vi "Run Test (ProjectRefnum).vi"(5 "Test Report":refnum<class "Test Report.lvclass">, 6 "Verbose":bool, 7 "Report Path":path, 8 "error in":errorcluster, 9 "Virtual Folder (My Computer)":string, 10 "Project Refnum":refnum<vi>, 11 "Interactive (T)":bool=TRUE) -> (0 "error out":errorcluster)   [LabVIEW 2013, in "Caraya.lvlib"]
uses:
  classes/Test Report/Test Report.lvclass
  Caraya.lvlib
  classes/Test Runner/Test Runner.lvclass
  classes/Test Runner.Project/Test Runner.Project.lvclass
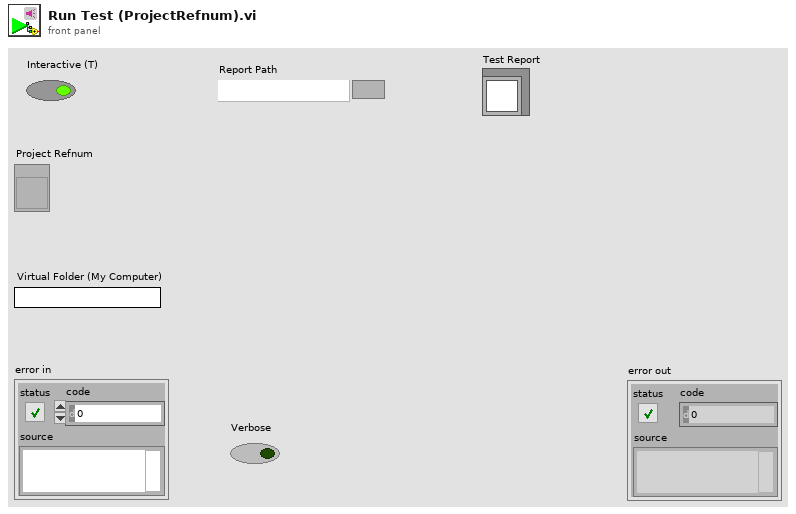
[diagram p1: front panel]
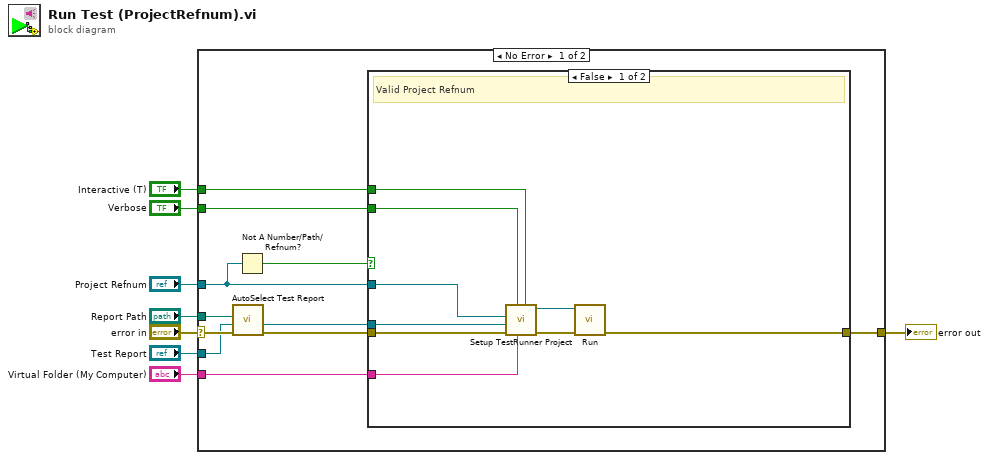
[diagram p0: block diagram]
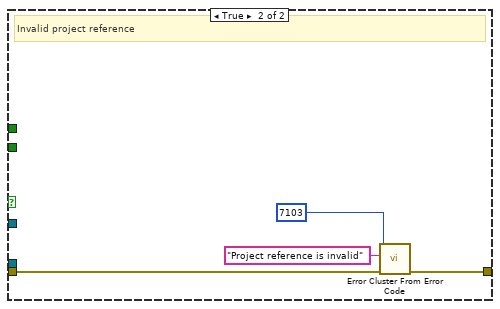
[diagram p2: hidden frame]
diagram:
  n1 = case shown="No Error" "error in" {
    selector: "error in" -> [w16 w33]
    tunnel: [w19 w33] -> w8
    tunnel: "Verbose" -> [w18 _]
    tunnel: "Interactive (T)" -> [w17 _]
    tunnel: "Test Report" -> [w13 _]
    tunnel: "Project Refnum" -> [w10 _]
    tunnel: "Report Path" -> [w15 _]
    tunnel: "Virtual Folder (My Computer)" -> [w11 _]
    frame No Error {
      n2 = call "AutoSelect Test Report.vi"("error in (no error)"=w16, "Test Report in"=w13, "Report Path"=w15) -> ("error out"=w14:errorcluster, "Test Report out"=w12:refnum<class "Test Report.lvclass">)  [unwired: 7 in]
      n3 = Not A Number/Path/Refnum?(number/path/refnum=w10) -> (NaN/Path/Refnum?=w9:bool)
      n4 = case shown="False" w9 {
        tunnel: [w28 w31] -> w19
        tunnel: w18 -> [w27 _]
        tunnel: w17 -> [w26 _]
        tunnel: w14 -> [w23 w32]
        tunnel: w12 -> [w22 _]
        tunnel: w11 -> [w21 _]
        tunnel: w10 -> [w20 _]
        frame False {
          # "Valid Project Refnum"
          n5 = call "Setup TestRunner Project.vi"("Interactive (T)"=w26, "Virtual Folder (empty: \"My Computer\")"=w21, "Verbose (F)"=w27, "error in (no error)"=w23, "Test Report"=w22, "Project Refnum"=w20) -> ("error out"=w24:errorcluster, "Test Runner.Project out"=w25:refnum<class "Test Runner.Project.lvclass">)  [unwired: 4 in]
          n6 = call "Run.vi"("error in (no error)"=w24, "Test Runner in"=w25) -> ("error out"=w28:errorcluster)  [unwired: 8 in, 1 out]
        }
        frame True {
          # "Invalid project reference"
          n7 = call <vilib>:"Error Cluster From Error Code.vi"("error in (no error)"=w32, "error message (\"\")"="Project reference is invalid" ("error message (\"\")"), "error code (0)"=7103 ("code")) -> ("error out"=w31:errorcluster)  [unwired: 6 in]
        }
      }
    }
    frame Error {
    }
  }
  "error out" <- w8
